vi "Autonomous State Machine RC.vi"   [LabVIEW 2014]
doc: "This VI is called when autonomous begins, and will automatically be terminated when autonomous ends. You can carry out timed or sensor driven robot movement independently without needing to return to the caller."
uses:
  <vilib>/Rock Robotics/WPI/RobotDrive/WPI_RobotDriveGetSetRefNum.vi
panel:
  # "Be sure to right-click and choose Data Operations>>Make Current Value default if you want to save the array values with the VI"
types:
  T1 = typedef "WPI_MotorControlDeviceRef.ctl" = cluster{"DeviceStatus":errorcluster, "Type":T2, "PWM":cluster{"Controller":T3, "PWM Channel":T4, "DeadBand":T5}, "CAN":cluster{"Device Number":u8, "Control Mode":T6, "Semaphore":T7, "Max Vout":dbl, "TalonSRX Control Mode":T8}, "Invert":bool, "TransformRef":T9, "InvTransformRef":T9}
  T2 = typedef "WPI_MotorControlType.ctl" = enum16{"PWM", "CAN", "CANTalonSRX"}
  T3 = typedef "FPGA_TypedefDigitalModule.ctl" = enum16{"Controller 1"}
  T4 = typedef "FPGA_DIOPWMChannel.ctl" = enum8{"PWM 0", "PWM 1", "PWM 2", "PWM 3", "PWM 4", "PWM 5", "PWM 6", "PWM 7", "PWM 8", "PWM 9", "PWM MXP 0", "PWM MXP 1", "PWM MXP 2", "PWM MXP 3", "PWM MXP 4", "PWM MXP 5", "PWM MXP 6", "PWM MXP 7", "PWM MXP 8", "PWM MXP 9", "Invalid"}
  T5 = typedef "WPI_PWMDeadband.ctl" = cluster{"Name":string, "maxPositivePwm":i32, "minPositivePwm":i32, "centerPwm":i32, "maxNegativePwm":i32, "minNegativePwm":i32, "angularRange":u16}
  T6 = typedef "WPI_CANJaguar_ControlMode.ctl" = enum8{"Percent VBus", "Current", "Speed", "Position", "Voltage"}
  T7 = typedef "Semaphore RefNum" = refnum<k1>
  T8 = typedef "WPI_CANTalonSRX_APIControlMode.ctl" = enum8{"Percent VBus", "Speed", "Position", "Slave", "Unchanged / Invalid"}
  T9 = typedef "WPI_PWMTransform_ConPane.ctl" = refnum<vi>
  T10 = typedef "WPI_CANTalonSRX_GlobalStatus.ctl" = cluster{"Applied Throttle":dbl, "Module Enabled":bool, "CAN Error":errorcluster, "Closed Loop Error":dbl, "Forward Limit Switch Closed":bool, "Reverse Limit Switch Closed":bool, "Sensor Position":dbl, "Sensor Velocity":dbl, "Current":dbl, "Sticky Fault - Over Temp":bool, "Sticky Fault - Under Voltage":bool, "Sticky Fault - Forward Limit":bool, "Sticky Fault - Reverse Limit":bool, "Sticky Fault - Forward Soft Limit":bool, "Sticky Fault - Reverse Soft Limit":bool, "Brake is Enabled":bool, "Encoder Position":dbl, "Encoder Velocity":dbl, "Encoder Index Count":dbl, "Encoder A Pin State":bool, "Encoder B Pin State":bool, "Encoder Index Pin State":bool, "Analog In":dbl, "Analog In Velocity":dbl, "Temperature (C)":dbl, "Battery Voltage":dbl}
  T11 = typedef "WPI_EncoderDevRef.ctl" = cluster{"DevStatus":errorcluster, "EncoderIndex":T12, "CounterIndex":T13, "DistancePerCount":dbl, "Decoding Type":T14}
  T12 = typedef "FPGA_EncoderIdx.ctl" = enum8{"Enc 0", "Enc 1", "Enc 2", "Enc 3", "Enc 4", "Enc 5", "Enc 6", "Enc 7", "Invalid"}
  T13 = typedef "FPGA_CounterCtrSystemIndex.ctl" = enum8{"Ctr 0", "Ctr 1", "Ctr 2", "Ctr 3", "Ctr 4", "Ctr 5", "Ctr 6", "Ctr 7", "Invalid"}
  T14 = typedef "WPI_EncoderType.ctl" = enum16{"1x", "2x", "4x"}
  T15 = typedef "WPI_RobotDriveDevRef.ctl" = cluster{"DevStatus":errorcluster, "Motors[]":T1[], "Square Inputs":bool, "Max Output":dbl}
  T16 = typedef "WPI_SwitchDevRef.ctl" = cluster{"DevStatus":errorcluster, "DIO Channel":T17, "Controller":T3, "CntIndex":T13, "Normally Closed":bool}
  T17 = typedef "FPGA_DIOChannel.ctl" = enum8{"DIO 0", "DIO 1", "DIO 2", "DIO 3", "DIO 4", "DIO 5", "DIO 6", "DIO 7", "DIO 8", "DIO 9", "DIO MXP 0", "DIO MXP 1", "DIO MXP 2", "DIO MXP 3", "DIO MXP 4", "DIO MXP 5", "DIO MXP 6", "DIO MXP 7", "DIO MXP 8", "DIO MXP 9", "DIO MXP 10", "DIO MXP 11", "DIO MXP 12", "DIO MXP 13", "DIO MXP 14", "DIO MXP 15", "Invalid"}
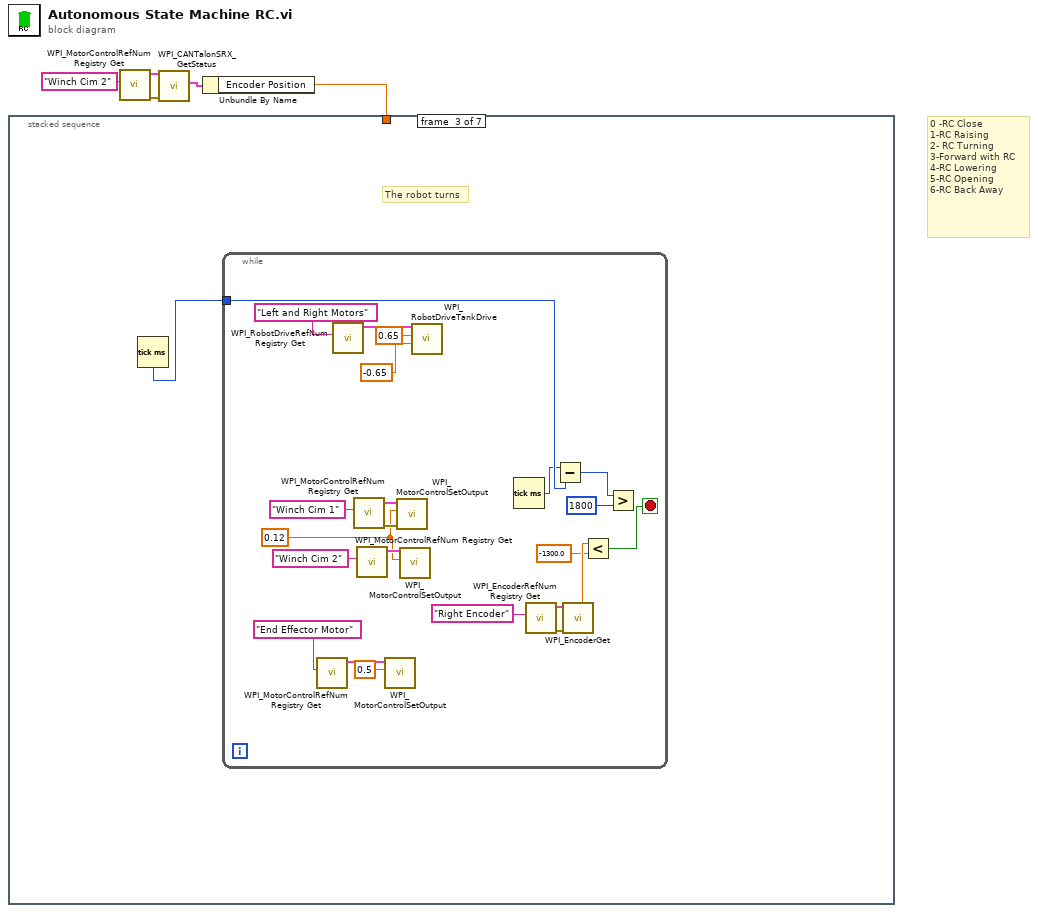
[diagram p0: block diagram]
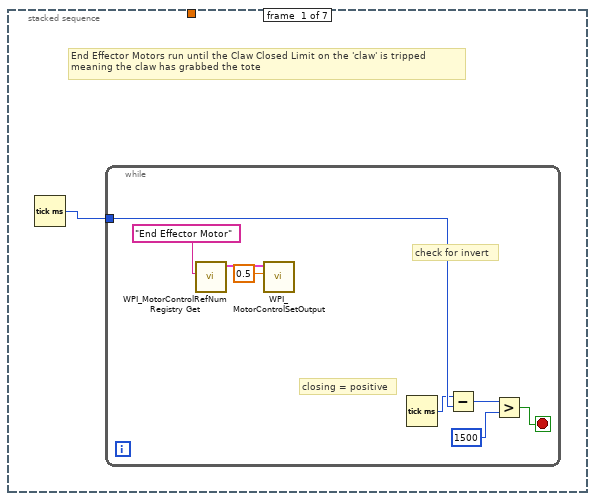
[diagram p2: hidden frame]
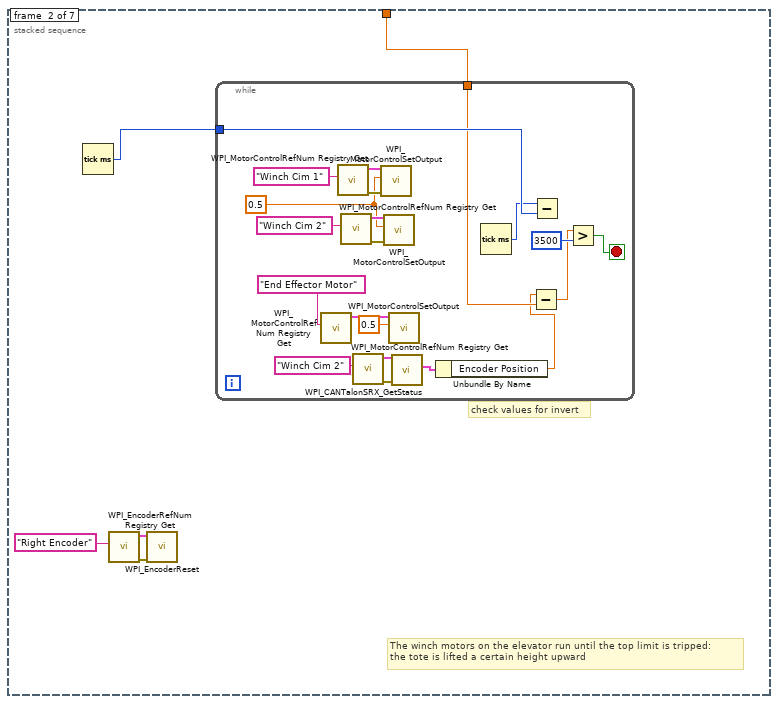
[diagram p3: hidden frame]
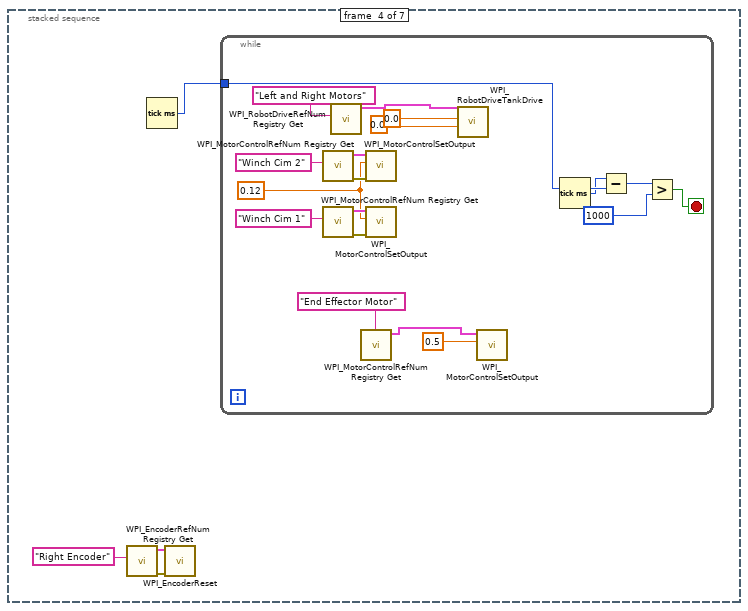
[diagram p4: hidden frame]
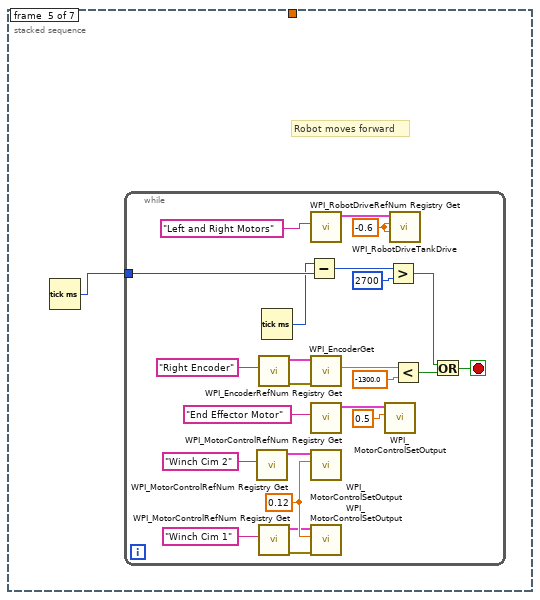
[diagram p5: hidden frame]
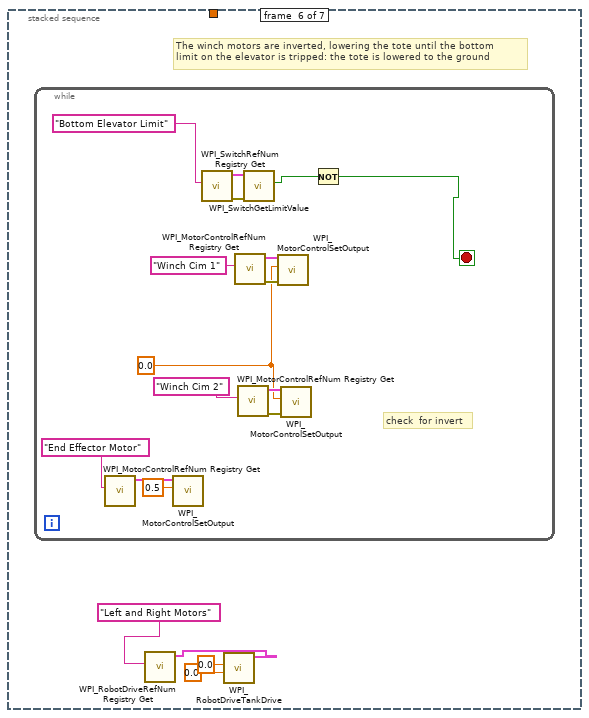
[diagram p6: hidden frame]
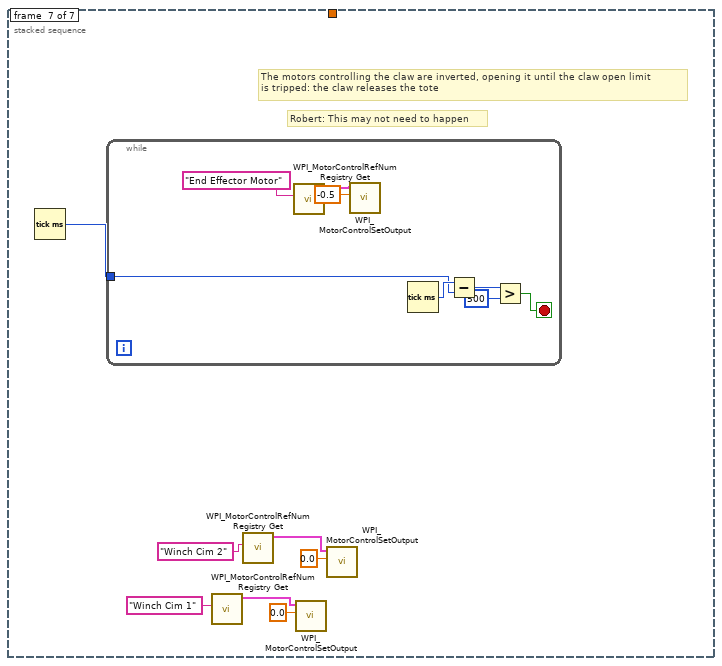
[diagram p7: hidden frame]
diagram:
  # "0 -RC Close\n1-RC Raising\n2- RC Turning\n3-Forward with RC\n4-RC Lowering\n5-RC Opening\n6-RC Back Away"
  n1 = call <vilib>:"WPI_MotorControlRefNum Registry Get.vi"("refnum name"="Winch Cim 2") -> ("error out"=w3:errorcluster, "MotorControlDevRef"=w4:T1)  [unwired: 9 in]
  n2 = call <vilib>:"WPI_CANTalonSRX_GetStatus.vi"("error in (no error)"=w3, "CAN Talon SRX Ref"=w4) -> ("Talon SRX Status"=w5:T10)  [unwired: 7 in, 2 out]
  n3 = Unbundle By Name(w5) -> ("Encoder Position"=w1:dbl)
  n4 = stacked-sequence {
    tunnel: w1 -> [_ w18 _ _ _ _ _]
    frame #0 {
      # "End Effector Motors run until the Claw Closed Limit on the 'claw' is tripped\nmeaning the claw has grabbed the tote"
      n5 = Tick Count (ms)() -> (millisecond timer value=w6:u32)
      n6 = while {
        tunnel: w6 -> [w11]
        stop <- w12 stop-if-true
        # "closing = positive"
        # "check for invert"
        n7 = call <vilib>:"WPI_MotorControlRefNum Registry Get.vi"("refnum name"="End Effector Motor") -> ("MotorControlDevRef"=w7:T1)  [unwired: 9 in, 1 out]
        n8 = call <vilib>:"WPI_MotorControlSetOutput.vi"("Output"=0.5, "MotorControlDevRef"=w7) -> ()  [unwired: 7 in, 3 out]
        n9 = Tick Count (ms)() -> (millisecond timer value=w10:u32)
        n10 = Subtract(x=w10, y=w11) -> (x-y=w14:u32)
        n11 = Greater?(x=w14, y=u32 1500) -> (0:w12:bool)
      }
    }
    frame #1 {
      # "The winch motors on the elevator run until the top limit is tripped: \nthe tote is lifted a certain height upward"
      # "check values for invert"
      n12 = Tick Count (ms)() -> (millisecond timer value=w19:u32)
      n13 = call <vilib>:"WPI_EncoderRefNum Registry Get.vi"("refnum name"="Right Encoder") -> ("error out"=w16:errorcluster, "EncoderDevRef"=w15:T11)  [unwired: 9 in]
      n14 = call <vilib>:"WPI_EncoderReset.vi"("error in (no error)"=w16, "EncoderDevRef"=w15) -> ()  [unwired: 8 in, 2 out]
      n15 = while {
        tunnel: w19 -> [w38]
        tunnel: w18 -> [w21]
        stop <- w39 stop-if-true
        w30 = 0.5
        n16 = call <vilib>:"WPI_MotorControlRefNum Registry Get.vi"("refnum name"="End Effector Motor") -> ("MotorControlDevRef"=w27:T1)  [unwired: 9 in, 1 out]
        n17 = call <vilib>:"WPI_MotorControlRefNum Registry Get.vi"("refnum name"="Winch Cim 1") -> ("error out"=w35:errorcluster, "MotorControlDevRef"=w34:T1)  [unwired: 9 in]
        n18 = call <vilib>:"WPI_MotorControlRefNum Registry Get.vi"("refnum name"="Winch Cim 2") -> ("error out"=w32:errorcluster, "MotorControlDevRef"=w31:T1)  [unwired: 9 in]
        n19 = call <vilib>:"WPI_MotorControlRefNum Registry Get.vi"("refnum name"="Winch Cim 2") -> ("error out"=w25:errorcluster, "MotorControlDevRef"=w24:T1)  [unwired: 9 in]
        n20 = call <vilib>:"WPI_MotorControlSetOutput.vi"("error in (no error)"=w35, "Output"=w30, "MotorControlDevRef"=w34) -> ()  [unwired: 6 in, 3 out]
        n21 = call <vilib>:"WPI_MotorControlSetOutput.vi"("error in (no error)"=w32, "Output"=w30, "MotorControlDevRef"=w31) -> ()  [unwired: 6 in, 3 out]
        n22 = call <vilib>:"WPI_MotorControlSetOutput.vi"("Output"=0.5, "MotorControlDevRef"=w27) -> ()  [unwired: 7 in, 3 out]
        n23 = call <vilib>:"WPI_CANTalonSRX_GetStatus.vi"("error in (no error)"=w25, "CAN Talon SRX Ref"=w24) -> ("Talon SRX Status"=w23:T10)  [unwired: 7 in, 2 out]
        n24 = Unbundle By Name(w23) -> ("Encoder Position"=w20:dbl)
        n25 = Tick Count (ms)() -> (millisecond timer value=w37:u32)
        n26 = Subtract(x=w20, y=w21) -> (x-y=w22:dbl)
        n27 = Subtract(x=w37, y=w38) -> ()  [unwired: 1 out]
        n28 = Greater?(x=w22, y=u32 3500) -> (0:w39:bool)
      }
    }
    frame #2 {
      # "The robot turns"
      n29 = Tick Count (ms)() -> (millisecond timer value=w41:u32)
      n30 = while {
        tunnel: w41 -> [w64]
        stop <- w42 stop-if-true
        w54 = 0.12
        n31 = call <vilib>:"WPI_MotorControlRefNum Registry Get.vi"("refnum name"="End Effector Motor") -> ("MotorControlDevRef"=w50:T1)  [unwired: 9 in, 1 out]
        n32 = call <vilib>:"WPI_RobotDriveRefNum Registry Get.vi"("refnum name"="Left and Right Motors") -> ("RobotDriveDevRef"=w62:T15)  [unwired: 9 in, 1 out]
        n33 = call <vilib>:"WPI_MotorControlRefNum Registry Get.vi"("refnum name"="Winch Cim 1") -> ("error out"=w57:errorcluster, "MotorControlDevRef"=w53:T1)  [unwired: 9 in]
        n34 = call <vilib>:"WPI_MotorControlRefNum Registry Get.vi"("refnum name"="Winch Cim 2") -> ("MotorControlDevRef"=w55:T1)  [unwired: 9 in, 1 out]
        n35 = call <vilib>:"WPI_MotorControlSetOutput.vi"("Output"=0.5, "MotorControlDevRef"=w50) -> ()  [unwired: 7 in, 3 out]
        n36 = call <vilib>:"WPI_MotorControlSetOutput.vi"("error in (no error)"=w57, "Output"=w54, "MotorControlDevRef"=w53) -> ()  [unwired: 6 in, 3 out]
        n37 = call <vilib>:"WPI_MotorControlSetOutput.vi"("Output"=w54, "MotorControlDevRef"=w55) -> ()  [unwired: 7 in, 3 out]
        n38 = call <vilib>:"WPI_RobotDriveTankDrive.vi"("Right axis value"=-0.65, "Left axis value"=0.65, "RobotDriveDevRef"=w62) -> ()  [unwired: 6 in, 3 out]
        n39 = Tick Count (ms)() -> (millisecond timer value=w63:u32)
        n40 = call <vilib>:"WPI_EncoderRefNum Registry Get.vi"("refnum name"="Right Encoder") -> ("error out"=w48:errorcluster, "EncoderDevRef"=w47:T11)  [unwired: 9 in]
        n41 = Subtract(x=w63, y=w64) -> (x-y=w44:u32)
        n42 = call <vilib>:"WPI_EncoderGet.vi"("error in (no error)"=w48, "EncoderDevRef"=w47) -> ("Distance"=w46:dbl)  [unwired: 4 in, 5 out]
        n43 = Less?(x=w46, y=-1300.0) -> (x < y?=w42:bool)
        n44 = Greater?(x=w44, y=u32 1800) -> ()  [unwired: 1 out]
      }
    }
    frame #3 {
      n45 = call <vilib>:"WPI_EncoderRefNum Registry Get.vi"("refnum name"="Right Encoder") -> ("error out"=w66:errorcluster, "EncoderDevRef"=w65:T11)  [unwired: 9 in]
      n46 = Tick Count (ms)() -> (millisecond timer value=w68:u32)
      n47 = call <vilib>:"WPI_EncoderReset.vi"("error in (no error)"=w66, "EncoderDevRef"=w65) -> ()  [unwired: 8 in, 2 out]
      n48 = while {
        tunnel: w68 -> [w85]
        stop <- w86 stop-if-true
        w73 = 0.12
        n49 = call <vilib>:"WPI_MotorControlRefNum Registry Get.vi"("refnum name"="Winch Cim 2") -> ("error out"=w75:errorcluster, "MotorControlDevRef"=w74:T1)  [unwired: 9 in]
        n50 = call <vilib>:"WPI_MotorControlRefNum Registry Get.vi"("refnum name"="Winch Cim 1") -> ("error out"=w78:errorcluster, "MotorControlDevRef"=w77:T1)  [unwired: 9 in]
        n51 = call <vilib>:"WPI_RobotDriveRefNum Registry Get.vi"("refnum name"="Left and Right Motors") -> ("RobotDriveDevRef"=w83:T15)  [unwired: 9 in, 1 out]
        n52 = call <vilib>:"WPI_MotorControlRefNum Registry Get.vi"("refnum name"="End Effector Motor") -> ("MotorControlDevRef"=w70:T1)  [unwired: 9 in, 1 out]
        n53 = call <vilib>:"WPI_MotorControlSetOutput.vi"("error in (no error)"=w75, "Output"=w73, "MotorControlDevRef"=w74) -> ()  [unwired: 6 in, 3 out]
        n54 = call <vilib>:"WPI_MotorControlSetOutput.vi"("error in (no error)"=w78, "Output"=w73, "MotorControlDevRef"=w77) -> ()  [unwired: 6 in, 3 out]
        n55 = call <vilib>:"WPI_RobotDriveTankDrive.vi"("Right axis value"=0.0, "Left axis value"=0.0, "RobotDriveDevRef"=w83) -> ()  [unwired: 6 in, 3 out]
        n56 = call <vilib>:"WPI_MotorControlSetOutput.vi"("Output"=0.5, "MotorControlDevRef"=w70) -> ()  [unwired: 7 in, 3 out]
        n57 = Tick Count (ms)() -> (millisecond timer value=w84:u32)
        n58 = Subtract(x=w84, y=w85) -> (x-y=w87:u32)
        n59 = Greater?(x=w87, y=1000) -> (0:w86:bool)
      }
    }
    frame #4 {
      # "Robot moves forward"
      n60 = Tick Count (ms)() -> (millisecond timer value=w88:u32)
      n61 = while {
        tunnel: w88 -> [w110]
        stop <- w89 stop-if-true
        w101 = 0.12
        w106 = -0.6 ("Left axis value")
        n62 = call <vilib>:"WPI_MotorControlRefNum Registry Get.vi"("refnum name"="Winch Cim 2") -> ("MotorControlDevRef"=w102:T1)  [unwired: 9 in, 1 out]
        n63 = call <vilib>:"WPI_EncoderRefNum Registry Get.vi"("refnum name"="Right Encoder") -> ("error out"=w95:errorcluster, "EncoderDevRef"=w94:T11)  [unwired: 9 in]
        n64 = call <vilib>:"WPI_MotorControlRefNum Registry Get.vi"("refnum name"="Winch Cim 1") -> ("error out"=w104:errorcluster, "MotorControlDevRef"=w100:T1)  [unwired: 9 in]
        n65 = Tick Count (ms)() -> (millisecond timer value=w109:u32)
        n66 = Subtract(x=w109, y=w110) -> (x-y=w112:u32)
        n67 = call <vilib>:"WPI_RobotDriveRefNum Registry Get.vi"("refnum name"="Left and Right Motors") -> ("RobotDriveDevRef"=w108:T15)  [unwired: 9 in, 1 out]
        n68 = call <vilib>:"WPI_EncoderGet.vi"("error in (no error)"=w95, "EncoderDevRef"=w94) -> ("Distance"=w93:dbl)  [unwired: 4 in, 5 out]
        n69 = call <vilib>:"WPI_MotorControlRefNum Registry Get.vi"("refnum name"="End Effector Motor") -> ("MotorControlDevRef"=w97:T1)  [unwired: 9 in, 1 out]
        n70 = call <vilib>:"WPI_MotorControlSetOutput.vi"("Output"=w101, "MotorControlDevRef"=w102) -> ()  [unwired: 7 in, 3 out]
        n71 = call <vilib>:"WPI_MotorControlSetOutput.vi"("error in (no error)"=w104, "Output"=w101, "MotorControlDevRef"=w100) -> ()  [unwired: 6 in, 3 out]
        n72 = call <vilib>:"WPI_MotorControlSetOutput.vi"("Output"=0.5, "MotorControlDevRef"=w97) -> ()  [unwired: 7 in, 3 out]
        n73 = Greater?(x=w112, y=u32 2700) -> (0:w90:bool)
        n74 = call <vilib>:"WPI_RobotDriveTankDrive.vi"("Right axis value"=w106, "Left axis value"=w106, "RobotDriveDevRef"=w108) -> ()  [unwired: 6 in, 3 out]
        n75 = Less?(x=w93, y=-1300.0) -> (x < y?=w91:bool)
        n76 = Or(x=w90, y=w91) -> (x .or. y?=w89:bool)
      }
    }
    frame #5 {
      # "The winch motors are inverted, lowering the tote until the bottom \nlimit on the elevator is tripped: the tote is lowered to the ground"
      n77 = while {
        stop <- w120 stop-if-true
        w125 = 0.0
        # "check  for invert"
        n78 = call <vilib>:"WPI_MotorControlRefNum Registry Get.vi"("refnum name"="End Effector Motor") -> ("MotorControlDevRef"=w117:T1)  [unwired: 9 in, 1 out]
        n79 = call <vilib>:"WPI_MotorControlSetOutput.vi"("Output"=0.5, "MotorControlDevRef"=w117) -> ()  [unwired: 7 in, 3 out]
        n80 = call <vilib>:"WPI_SwitchRefNum Registry Get.vi"("refnum name"="Bottom Elevator Limit") -> ("error out"=w124:errorcluster, "SwitchDevRef"=w123:T16)  [unwired: 9 in]
        n81 = call <vilib>:"WPI_MotorControlRefNum Registry Get.vi"("refnum name"="Winch Cim 1") -> ("error out"=w130:errorcluster, "MotorControlDevRef"=w129:T1)  [unwired: 9 in]
        n82 = call <vilib>:"WPI_MotorControlRefNum Registry Get.vi"("refnum name"="Winch Cim 2") -> ("error out"=w127:errorcluster, "MotorControlDevRef"=w126:T1)  [unwired: 9 in]
        n83 = call <vilib>:"WPI_SwitchGetLimitValue.vi"("error in (no error)"=w124, "SwitchDevRef"=w123) -> ("Switch Pressed"=w121:bool)  [unwired: 7 in, 2 out]
        n84 = call <vilib>:"WPI_MotorControlSetOutput.vi"("error in (no error)"=w130, "Output"=w125, "MotorControlDevRef"=w129) -> ()  [unwired: 6 in, 3 out]
        n85 = call <vilib>:"WPI_MotorControlSetOutput.vi"("error in (no error)"=w127, "Output"=w125, "MotorControlDevRef"=w126) -> ()  [unwired: 6 in, 3 out]
        n86 = Not(x=w121) -> (.not. x?=w120:bool)
      }
      n87 = call <vilib>:"WPI_RobotDriveRefNum Registry Get.vi"("refnum name"="Left and Right Motors") -> ("RobotDriveDevRef"=w116:T15)  [unwired: 9 in, 1 out]
      n88 = call <vilib>:"WPI_RobotDriveTankDrive.vi"("Right axis value"=0.0, "Left axis value"=0.0, "RobotDriveDevRef"=w116) -> ()  [unwired: 6 in, 3 out]
    }
    frame #6 {
      # "Robert: This may not need to happen"
      # "The motors controlling the claw are inverted, opening it until the claw open limit\nis tripped: the claw releases the tote"
      n89 = Tick Count (ms)() -> (millisecond timer value=w138:u32)
      n90 = while {
        tunnel: w138 -> [w139]
        stop <- w144 stop-if-true
        n91 = call <vilib>:"WPI_MotorControlRefNum Registry Get.vi"("refnum name"="End Effector Motor") -> ("MotorControlDevRef"=w141:T1)  [unwired: 9 in, 1 out]
        n92 = call <vilib>:"WPI_MotorControlSetOutput.vi"("Output"=-0.5, "MotorControlDevRef"=w141) -> ()  [unwired: 7 in, 3 out]
        n93 = Tick Count (ms)() -> (millisecond timer value=w143:u32)
        n94 = Subtract(x=w143, y=w139) -> (x-y=w146:u32)
        n95 = Greater?(x=w146, y=u32 500) -> (0:w144:bool)
      }
      n96 = call <vilib>:"WPI_MotorControlRefNum Registry Get.vi"("refnum name"="Winch Cim 1") -> ("MotorControlDevRef"=w133:T1)  [unwired: 9 in, 1 out]
      n97 = call <vilib>:"WPI_MotorControlRefNum Registry Get.vi"("refnum name"="Winch Cim 2") -> ("MotorControlDevRef"=w136:T1)  [unwired: 9 in, 1 out]
      n98 = call <vilib>:"WPI_MotorControlSetOutput.vi"("Output"=0.0, "MotorControlDevRef"=w133) -> ()  [unwired: 7 in, 3 out]
      n99 = call <vilib>:"WPI_MotorControlSetOutput.vi"("Output"=0.0, "MotorControlDevRef"=w136) -> ()  [unwired: 7 in, 3 out]
    }
  }
